vi "Start Autofocus.vi"(8 "error in (no error)":errorcluster, 10 "Camera Settings":T1={"Exposure Time (ms)"=100.0, "Binning"=enum."2x2", "Scan Mode"=0, "Frames to Acquire"=1000.0, "Pixel Correction"=TRUE, "Frames to Skip"=0, "File Path"=path "", "Duty cycle"=0.2, "ALEX"=FALSE, "Shutter Enable"=[], "Timelapse Interval (s)"=0} {"Timelapse Interval (s)" max=60000 step=1; "Exposure Time (ms)" min=1.0 max=10000.0 step=1.0}, 11 "Application in":refnum<class "Application.lvclass">) -> (0 "error out":errorcluster, 3 "Application out":refnum<class "Application.lvclass">)   [LabVIEW 2018, in "Application.lvlib" / "Application.lvclass"]
uses:
  Application.lvclass
  Resources/Type Defs/Camera Settings.ctl
  Application.lvclass/Application.ctl
  Mode.ctl
  <vilib>/ActorFramework/Message Enqueuer/Message Enqueuer.lvclass/Message Enqueuer.ctl
  <vilib>/ActorFramework/Message Enqueuer/Enqueue.vi
  Hardware/Stage Controller Messages/Start Autofocus Msg/Start Autofocus Msg.lvclass
  C:/Program Files/National Instruments/LabVIEW 2018/vi.lib/ActorFramework/Message/Message.lvclass
  <vilib>/ActorFramework/Message Priority Queue/Priority Enqueue.vi
  Application.lvlib
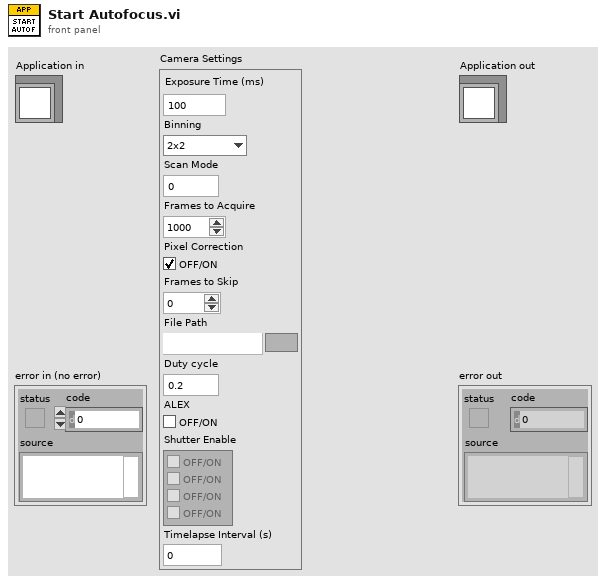
[diagram p1: front panel]
types:
  T1 = typedef "Camera Settings.ctl" = cluster{"Exposure Time (ms)":dbl, "Binning":enum16{"1x1", "2x2", "4x4"}, "Scan Mode":i32, "Frames to Acquire":dbl, "Pixel Correction":bool, "Frames to Skip":u32, "File Path":path, "Duty cycle":dbl, "ALEX":bool, "Shutter Enable":bool[], "Timelapse Interval (s)":u32}
  T2 = typedef "Application.lvlib/Mode.ctl" = enum16{"Idle", "Live", "Stream", "Autofocus", "Z-Stack"}
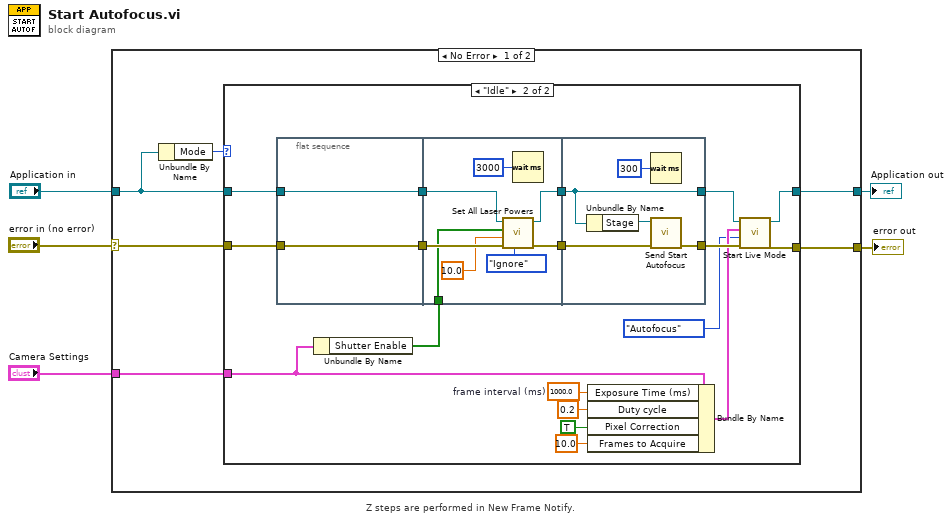
[diagram p0: block diagram]
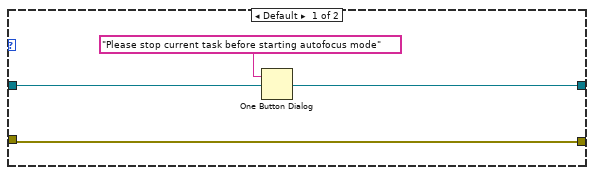
[diagram p2: hidden frame]
diagram:
  # "Z steps are performed in New Frame Notify."
  n1 = case shown="No Error" "error in (no error)" {
    selector: "error in (no error)" -> [w8 w49]
    tunnel: [w11 w49] -> w4
    tunnel: "Application in" -> [w7 w48]
    tunnel: "Camera Settings" -> [w9 _]
    tunnel: [w10 w48] -> w1
    frame No Error {
      n2 = Unbundle By Name(w7) -> ("Mode"=w6:T2)
      n3 = case shown="\"Idle\"" w6 {
        tunnel: [w13 w25] -> w11
        tunnel: [w14 w26] -> w10
        tunnel: w9 -> [_ w22]
        tunnel: w8 -> [w13 w28]
        tunnel: w7 -> [w14 w20]
        frame Default {
          n4 = One Button Dialog(message="Please stop current task before starting autofocus mode") -> ()  [unwired: 1 in, 1 out]
        }
        frame "Idle" {
          w29 = 1000.0  # frame interval (ms)
          n5 = flat-sequence {
            tunnel: w20 -> [w33]
            tunnel: w28 -> [w34]
            tunnel: [w34] -> w16
            tunnel: [w33] -> w15
            tunnel: [w40] -> w23
            tunnel: w21 -> [w39]
            tunnel: [w35] -> w19
            tunnel: w16 -> [w41]
            tunnel: w15 -> [w36]
            tunnel: [w46] -> w32
            tunnel: w23 -> [w45]
            tunnel: w19 -> [w44]
            tunnel: [w44] -> w18
            frame #0 {
            }
            frame #1 {
              n6 = call-dynamic "Set All Laser Powers.vi"("Mode"=enum16{"Normal", "Ignore", "Reset"}."Ignore", "error in (no error)"=w41, "Power"=10.0, "Line Enable"=w39, "Application in"=w36) -> ("error out"=w40:errorcluster, "Application out"=w35:refnum<class "Application.lvclass">)  [unwired: 5 in]
              n7 = Wait (ms)(milliseconds to wait=u32 3000) -> ()  [unwired: 1 out]
            }
            frame #2 {
              n8 = Unbundle By Name(w44) -> ("Stage"=w43:refnum<class "Message Enqueuer.lvclass">)
              n9 = Wait (ms)(milliseconds to wait=u32 300) -> ()  [unwired: 1 out]
              n10 = call "Send Start Autofocus.vi"("error in (no error)"=w45, "Message Enqueuer"=w43) -> ("error out"=w46:errorcluster)  [unwired: 8 in, 1 out]
            }
          }
          n11 = Unbundle By Name(w22) -> ("Shutter Enable"=w21:bool[])
          n12 = Bundle By Name(cluster=w22, "Exposure Time (ms)"=w29, "Duty cycle"=0.2, "Pixel Correction"=TRUE, "Frames to Acquire"=10.0) -> (w31:T1)
          n13 = call-dynamic "Start Live Mode.vi"("error in (no error)"=w32, "Mode"=Mode."Autofocus", "Camera Settings"=w31, "Application in"=w18) -> ("error out"=w25:errorcluster, "Application out"=w26:refnum<class "Application.lvclass">)  [unwired: 6 in]
        }
      }
    }
    frame Error {
    }
  }
  "error out" <- w4
  "Application out" <- w1
